vi "Decimate Data Store.vi"(9 "Data Store":T2) -> (1 "Data Points":T4[][](array[typedef]), 2 "Timestamps":T1[][](array[typedef]))   [LabVIEW 2012, in "File IO.lvclass"]
uses:
  File IO.lvclass
  Instruments/Utility Classes/Readable/X.ctl
  Instruments/Utility Classes/Readable/Data Store.ctl
  Instruments/Utility Classes/Readable/Data Point.ctl
  Instruments/Utility Classes/Readable/Time.ctl
  Instruments/Utility Classes/Readable/Readable.lvclass
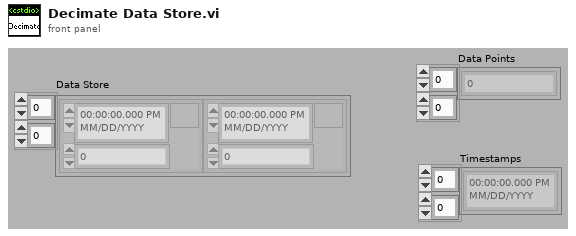
[diagram p1: front panel]
types:
  T1 = typedef "Readable.lvclass/Time.ctl" = timestamp
  T2 = typedef "Readable.lvclass/Data Store.ctl" = T3[][]
  T3 = typedef "Readable.lvclass/Data Point.ctl" = cluster{"t":T1, "x":T4}
  T4 = typedef "Readable.lvclass/X.ctl" = dbl
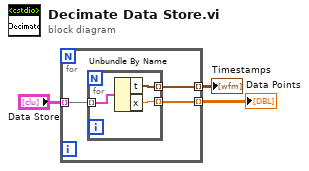
[diagram p0: block diagram]
diagram:
  n1 = for {
    tunnel: "Data Store" -> [w6] mode=indexing
    tunnel: [w5] -> w3 mode=indexing
    tunnel: [w4] -> w1 mode=indexing
    n2 = for {
      tunnel: w6 -> [w9] mode=indexing
      tunnel: [w8] -> w5 mode=indexing
      tunnel: [w7] -> w4 mode=indexing
      n3 = Unbundle By Name(w9) -> ("t"=w7:T1, "x"=w8:T4)
    }
  }
  "Data Points" <- w3
  "Timestamps" <- w1
